vi "default.vi"(8 "error in (no error)":errorcluster) -> (0 "error out":errorcluster)   [LabVIEW 2015, in "lv-config-json.lvlib"]
uses:
  lv-config-json.lvlib
  _controls/command.ctl
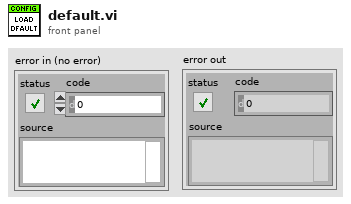
[diagram p1: front panel]
types:
  T1 = typedef "lv-config-json.lvlib/command.ctl" = enum16{"<commands>", "read_config", "write_config", "write_placeholder", "<null>"}
  T2 = typedef "lv-config-json.lvlib/master_config.ctl" = cluster{"placeholder":cluster{"random":dbl}}
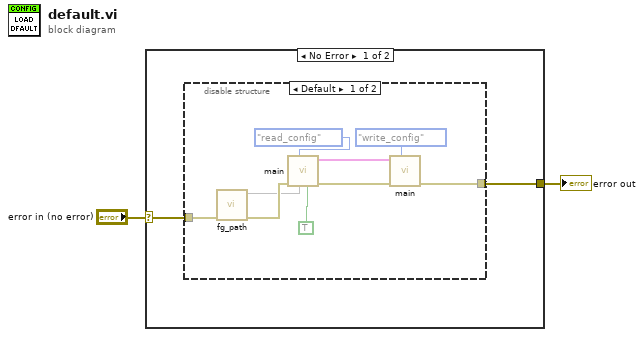
[diagram p0: block diagram]
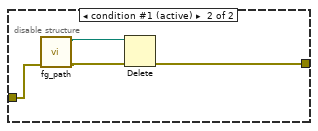
[diagram p2: hidden frame]
diagram:
  n1 = case shown="No Error" "error in (no error)" {
    selector: "error in (no error)" -> [w4 w18]
    tunnel: [w3 w18] -> w1
    frame No Error {
      n2 = disable-structure shown="Default" {
        disable-tunnel: w4 -> [w13 w14]
        disable-tunnel: [w7 w17] -> w3
        frame condition #0 {
          n3 = call "fg_path.vi"("error in (no error)"=w13) -> ("error out"=w12:errorcluster, 2:w11)  [unwired: 8 in, 1 out]
          n4 = call "main.vi"("force_read?"=TRUE, "custom_path"=w11, "command"=command."read_config" ("Config Commands"), "error in (no error)"=w12) -> ("error out"=w10:errorcluster, "config out"=w9:T2)  [unwired: 6 in]
          n5 = call "main.vi"("command"=command."write_config" ("Config Commands"), "error in (no error)"=w10, "config in"=w9) -> ("error out"=w7:errorcluster)  [unwired: 7 in, 1 out]
        }
        frame condition #1 (active) {
          n6 = call "fg_path.vi"("error in (no error)"=w14) -> ("error out"=w15:errorcluster, "config_working"=w16:path)  [unwired: 9 in]
          n7 = Delete(path (use dialog)=w16, error in=w15) -> (error out=w17:errorcluster)  [unwired: 3 in, 2 out]
        }
      }
    }
    frame Error {
    }
  }
  "error out" <- w1
